vi "MainIdent RT.vi"   [LabVIEW 2018]
doc: "The myRIO Project template acquires acceleration data from the onboard accelerometer and displays the changes of acceleration values in a waveform chart."
uses:
  <vilib>/myRIO/Common/Instrument Driver Framework/myRIO v1.0/Encoder/typedefs/Encoder Signal Mode.ctl
  <vilib>/Platform/TimedLoop/XDataNode/timing_clust.ctl
  <vilib>/Platform/TimedLoop/XDataNode/nitl_modes.ctl
  <vilib>/Platform/TimedLoop/XDataNode/wakeup.ctl
  <vilib>/myRIO/Instrument Drivers/Onboard IO/AI/typedefs/AI Reference.ctl
  <vilib>/myRIO/Common/Instrument Driver Framework/Utilities/typedefs/myRIO Generic Hardware Reference.ctl
  <vilib>/myRIO/Common/Instrument Driver Framework/Utilities/typedefs/Hardware Version Enum.ctl
  <vilib>/myRIO/Common/Instrument Driver Framework/Utilities/typedefs/myRIO v1.0 Reference.ctl
  <vilib>/myRIO/Common/Instrument Driver Framework/Utilities/typedefs/Generic FPGA Reference.ctl
  <vilib>/myRIO/Common/Instrument Driver Framework/myRIO v1.0/AI/typedefs/AI Channels List.ctl
  <vilib>/myRIO/Common/Instrument Driver Framework/myRIO v1.0/AI/typedefs/AI Channels Enum.ctl
  <vilib>/myRIO/Common/Instrument Driver Framework/Utilities/typedefs/Analog Scaling Constants List.ctl
  <vilib>/myRIO/Common/Instrument Driver Framework/Utilities/typedefs/Analog Scaling Constants.ctl
  <vilib>/userdefined/High Color/nirio_resource_hc.ctl
  <vilib>/myRIO/Instrument Drivers/Onboard IO/PWM/typedefs/PWM Reference.ctl
  <vilib>/myRIO/Common/Instrument Driver Framework/myRIO v1.0/PWM/typedefs/PWM Channels Enum.ctl
  <vilib>/myRIO/Instrument Drivers/Onboard IO/PWM/typedefs/PWM Configuration.ctl
  <vilib>/myRIO/Common/Instrument Driver Framework/myRIO v1.0/Encoder/typedefs/Encoder Configuration v1.0.ctl
  <vilib>/myRIO/Instrument Drivers/Onboard IO/Encoder/typedefs/Encoder Reference.ctl
  <vilib>/myRIO/Common/Instrument Driver Framework/myRIO v1.0/Encoder/typedefs/Encoder Channels Enum.ctl
  <vilib>/myRIO/Common/Instrument Driver Framework/myRIO v1.0/AI/vis/myRIO v1.1 Open AI.vi
  <vilib>/myRIO/Common/Instrument Driver Framework/myRIO v1.0/PWM/vis/myRIO v1.1 Open PWM.vi
  <vilib>/myRIO/Common/Instrument Driver Framework/myRIO v1.0/Encoder/vis/myRIO v1.1 Open Encoder.vi
  <vilib>/myRIO/Common/Instrument Driver Framework/Utilities/vis/Validate Channels.vi
  <vilib>/myRIO/Common/Instrument Driver Framework/myRIO v1.0/AI/vis/myRIO v1.0 Reserve AI.vi
  <vilib>/myRIO/Common/Instrument Driver Framework/myRIO v1.0/PWM/vis/myRIO v1.0 Reserve PWM.vi
  <vilib>/myRIO/Instrument Drivers/Onboard IO/PWM/vis/Set Duty Cycle and Frequency.vi
  <vilib>/myRIO/Common/Instrument Driver Framework/myRIO v1.0/Encoder/vis/myRIO v1.0 Reserve Encoder.vi
  <vilib>/myRIO/Common/Instrument Driver Framework/myRIO v1.0/Encoder/vis/myRIO v1.0 Close Encoder.vi
  <vilib>/myRIO/Common/Instrument Driver Framework/myRIO v1.0/PWM/vis/myRIO v1.0 Close PWM.vi
  <vilib>/myRIO/Common/Instrument Driver Framework/myRIO v1.0/AI/vis/myRIO v1.0 Build MUX Configuration AI.vi
  <vilib>/myRIO/Common/Instrument Driver Framework/myRIO v1.0/Resource Manager/vis/myRIO v1.0 Reserve Channel List.vi
  <vilib>/myRIO/Common/Instrument Driver Framework/myRIO v1.0/PWM/vis/myRIO v1.0 Build MUX Configuration PWM.vi
  <vilib>/myRIO/Common/Instrument Driver Framework/myRIO v1.0/Encoder/vis/myRIO v1.0 Build MUX Configuration Encoder.vi
  <vilib>/myRIO/Common/Instrument Driver Framework/myRIO v1.0/Encoder/vis/myRIO v1.0 Unreserve Encoder.vi
  <vilib>/myRIO/Common/Instrument Driver Framework/myRIO v1.0/PWM/vis/myRIO v1.0 Unreserve PWM.vi
  <vilib>/myRIO/Common/Instrument Driver Framework/myRIO v1.0/Resource Manager/vis/myRIO v1.0 Reserve Channel.vi
  <vilib>/myRIO/Common/Instrument Driver Framework/myRIO v1.0/Resource Manager/vis/myRIO v1.0 Unreserve Channel.vi
  <vilib>/myRIO/Common/Instrument Driver Framework/myRIO v1.0/Resource Manager/vis/myRIO v1.0 Create Configuration List.vi
  <vilib>/myRIO/Common/Instrument Driver Framework/myRIO v1.0/Resource Manager/vis/myRIO v1.0 Unreserve Channel List.vi
  <vilib>/myRIO/Common/Instrument Driver Framework/myRIO v1.0/Resource Manager/vis/myRIO v1.0 Build Mutex Name.vi
  <vilib>/Utility/VariantDataType/GetNumericInfo.vi
  <vilib>/Utility/error.llb/Error Cluster From Error Code.vi
  <vilib>/myRIO/Common/Instrument Driver Framework/myRIO v1.0/myRIO v1.1 Open.vi
  <vilib>/myRIO/Common/Instrument Driver Framework/Utilities/vis/IO Manager.vi
  <vilib>/myRIO/Common/Instrument Driver Framework/Utilities/vis/Configuration Manager.vi
  <vilib>/myRIO/Common/Instrument Driver Framework/myRIO v1.0/Resource Manager/vis/myRIO v1.0 Configure IO.vi
  <vilib>/myRIO/Common/Instrument Driver Framework/myRIO v1.0/myRIO v1.0 Close.vi
  <vilib>/myRIO/Common/Instrument Driver Framework/myRIO v1.0/PWM/vis/myRIO v1.0 Write PWM.vi
  <vilib>/myRIO/Common/Instrument Driver Framework/myRIO v1.0/Encoder/vis/myRIO v1.0 Configure Encoder.vi
  <vilib>/myRIO/Common/Instrument Driver Framework/myRIO v1.0/Encoder/vis/myRIO v1.0 Enable Encoder.vi
  <vilib>/myRIO/Common/Instrument Driver Framework/myRIO v1.0/AI/vis/myRIO v1.0 Get Scaling Constants AI.vi
  <vilib>/myRIO/Common/Instrument Driver Framework/myRIO v1.0/AI/vis/myRIO v1.0 Read AI.vi
  <vilib>/myRIO/Common/Instrument Driver Framework/myRIO v1.0/Encoder/vis/myRIO v1.0 Read Encoder.vi
  <vilib>/myRIO/Common/Instrument Driver Framework/myRIO v1.0/Encoder/vis/myRIO v1.0 Shutdown Encoder.vi
  <vilib>/myRIO/Common/Instrument Driver Framework/myRIO v1.0/PWM/vis/myRIO v1.0 Shutdown PWM.vi
  <vilib>/platform/TimedLoop/XDataNode/XDataNode.xnode
  <vilib>/myRIO/Instrument Drivers/Onboard IO/PWM/vis/myRIO PWM Open.xnode
  <vilib>/myRIO/Instrument Drivers/Onboard IO/Encoder/vis/myRIO Encoder Open.xnode
  <vilib>/myRIO/Instrument Drivers/Onboard IO/AI/vis/myRIO AI Open.xnode
  <vilib>/Platform/TimedLoop/XDataNode/XDNodeRunTimeDep.lvlib
  <vilib>/myRIO/Instrument Drivers/Onboard IO/Encoder/Encoder.lvlib
  <vilib>/myRIO/Instrument Drivers/Onboard IO/PWM/PWM.lvlib
  <vilib>/myRIO/Instrument Drivers/Onboard IO/AI/AI.lvlib
types:
  T1 = typedef "Encoder Signal Mode.ctl" = enum16{"Quadrature phase signal", "Step and direction signal"}
  T2 = typedef "AI.lvlib/AI Reference.ctl" = cluster{"myRIO Reference":T3, "AI Channels List":T7, "AI Scaling Constants List":T9}
  T3 = typedef "myRIO Generic Hardware Reference.ctl" = cluster{"myRIO Model":T4, "myRIO Hardware Reference":T5}
  T4 = typedef "Hardware Version Enum.ctl" = enum16{"Unknown", "myRIO-1900", "myRIO-1950", "roboRIO", "NI ELVIS RIO CM", "ELVIS III"}
  T5 = typedef "myRIO v1.0 Reference.ctl" = cluster{"Generic FPGA Reference":T6, "Allow multiple opens":bool}
  T6 = typedef "Generic FPGA Reference.ctl" = refnum<k20>
  T7 = typedef "AI Channels List.ctl" = T8[]
  T8 = typedef "AI Channels Enum.ctl" = enum16{"Not Connected", "AudioIn/Left", "AudioIn/Right", "C/AI0", "C/AI1", "A/AI0", "A/AI1", "A/AI2", "A/AI3", "A/AI4", "A/AI5", "A/AI6", "A/AI7", "B/AI0", "B/AI1", "B/AI2", "B/AI3", "B/AI4", "B/AI5", "B/AI6", "B/AI7", "AI/AI0", "AI/AI1", "AI/AI2", "AI/AI3", "A/AI0 (DIFF)", "A/AI1 (DIFF)", "A/AI2 (DIFF)", "A/AI3 (DIFF)", "B/AI0 (DIFF)", "B/AI1 (DIFF)", "B/AI2 (DIFF)", "B/AI3 (DIFF)"}
  T9 = typedef "Analog Scaling Constants List.ctl" = T10[]
  T10 = typedef "Analog Scaling Constants.ctl" = cluster{"LSB Weight (Volts)":dbl, "Offset (Volts)":dbl, "Signed?":bool}
  T11 = typedef "PWM.lvlib/PWM Reference.ctl" = cluster{"myRIO Reference":T3, "PWM Channels Enum":T12, "PWM Configuration":T13}
  T12 = typedef "PWM Channels Enum.ctl" = enum16{"Not Connected", "C/PWM0", "C/PWM1", "A/PWM0", "A/PWM1", "A/PWM2", "A/PWM3", "A/PWM4", "A/PWM5", "A/PWM6", "A/PWM7", "A/PWM8", "A/PWM9", "A/PWM10", "A/PWM11", "A/PWM12", "A/PWM13", "A/PWM14", "A/PWM15", "A/PWM16", "A/PWM17", "A/PWM18", "A/PWM19", "B/PWM0", "B/PWM1", "B/PWM2", "B/PWM3", "B/PWM4", "B/PWM5", "B/PWM6", "B/PWM7", "B/PWM8", "B/PWM9", "B/PWM10", "B/PWM11", "B/PWM12", "B/PWM13", "B/PWM14", "B/PWM15", "B/PWM16", "B/PWM17", "B/PWM18", "B/PWM19", "PWM/PWM0", "PWM/PWM1", "PWM/PWM2", "PWM/PWM3", "PWM/PWM4", "PWM/PWM5", "PWM/PWM6", "PWM/PWM7", "PWM/PWM8", "PWM/PWM9"}
  T13 = typedef "PWM.lvlib/PWM Configuration.ctl" = cluster{"Frequency":dbl, "Duty Cycle":dbl}
  T14 = typedef "Encoder.lvlib/Encoder Reference.ctl" = cluster{"myRIO Reference":T3, "Encoder Channels Enum":T15}
  T15 = typedef "Encoder Channels Enum.ctl" = enum16{"Not Connected", "C/ENC0", "C/ENC1", "A/ENC", "A/ENC0", "A/ENC1", "A/ENC2", "A/ENC3", "A/ENC4", "A/ENC5", "A/ENC6", "A/ENC7", "A/ENC8", "A/ENC9", "B/ENC", "B/ENC0", "B/ENC1", "B/ENC2", "B/ENC3", "B/ENC4", "B/ENC5", "B/ENC6", "B/ENC7", "B/ENC8", "B/ENC9", "DIO/ENC0", "DIO/ENC1", "DIO/ENC2", "DIO/ENC3", "DIO/ENC4"}
  T16 = typedef "XDNodeRunTimeDep.lvlib/timing_clust.ctl" = cluster{"Expected End [f-1]":u64, "Actual End [f-1]":u64, "Finished Late? [f-1]":bool, "Expected End [i-1]":u64, "Actual End [i-1]":u64, "Finished Late? [i-1]":bool, "Expected Start [i]":u64, "Actual Start [i]":u64, "Expected Start [f]":u64, "Actual Start [f]":u64, "Source Name":string, "Structure Name":string, "Period":i64, "Deadline":i64, "Offset":i64, "Start":i64, "Priority":i32, "Timeout":i32, "Mode":T17, "Wakeup Reason":T18, "Error":errorcluster, "Source Type":string, "Secondary Source Type":string, "Global End Time":u64, "Global Start Time":u64, "Frame Duration":u64, "Iteration Duration":u64, "Assigned CPU":i32, "I/O Scan Engine Mode":u32}
  T17 = typedef "XDNodeRunTimeDep.lvlib/nitl_modes.ctl" = enum32{"No Change", "Process missed periods, maintain original phase", "Discard missed periods, maintain original phase", "Process missed periods, ignore original phase", "Discard missed periods, ignore original phase"}
  T18 = typedef "XDNodeRunTimeDep.lvlib/wakeup.ctl" = enum32{"Normal", "Aborted", "Asynchronous wakeup", "Timing source error", "Timed loop error", "Timeout"}
  T19 = cluster{"dbl Scaled Value":dbl, dbl, "Double":dbl, "seconds since 1Jan1904":timestamp}
  T20 = cluster{"Double":dbl, "dbl Scaled Value":dbl, "Output":dbl, "seconds since 1Jan1904":timestamp}
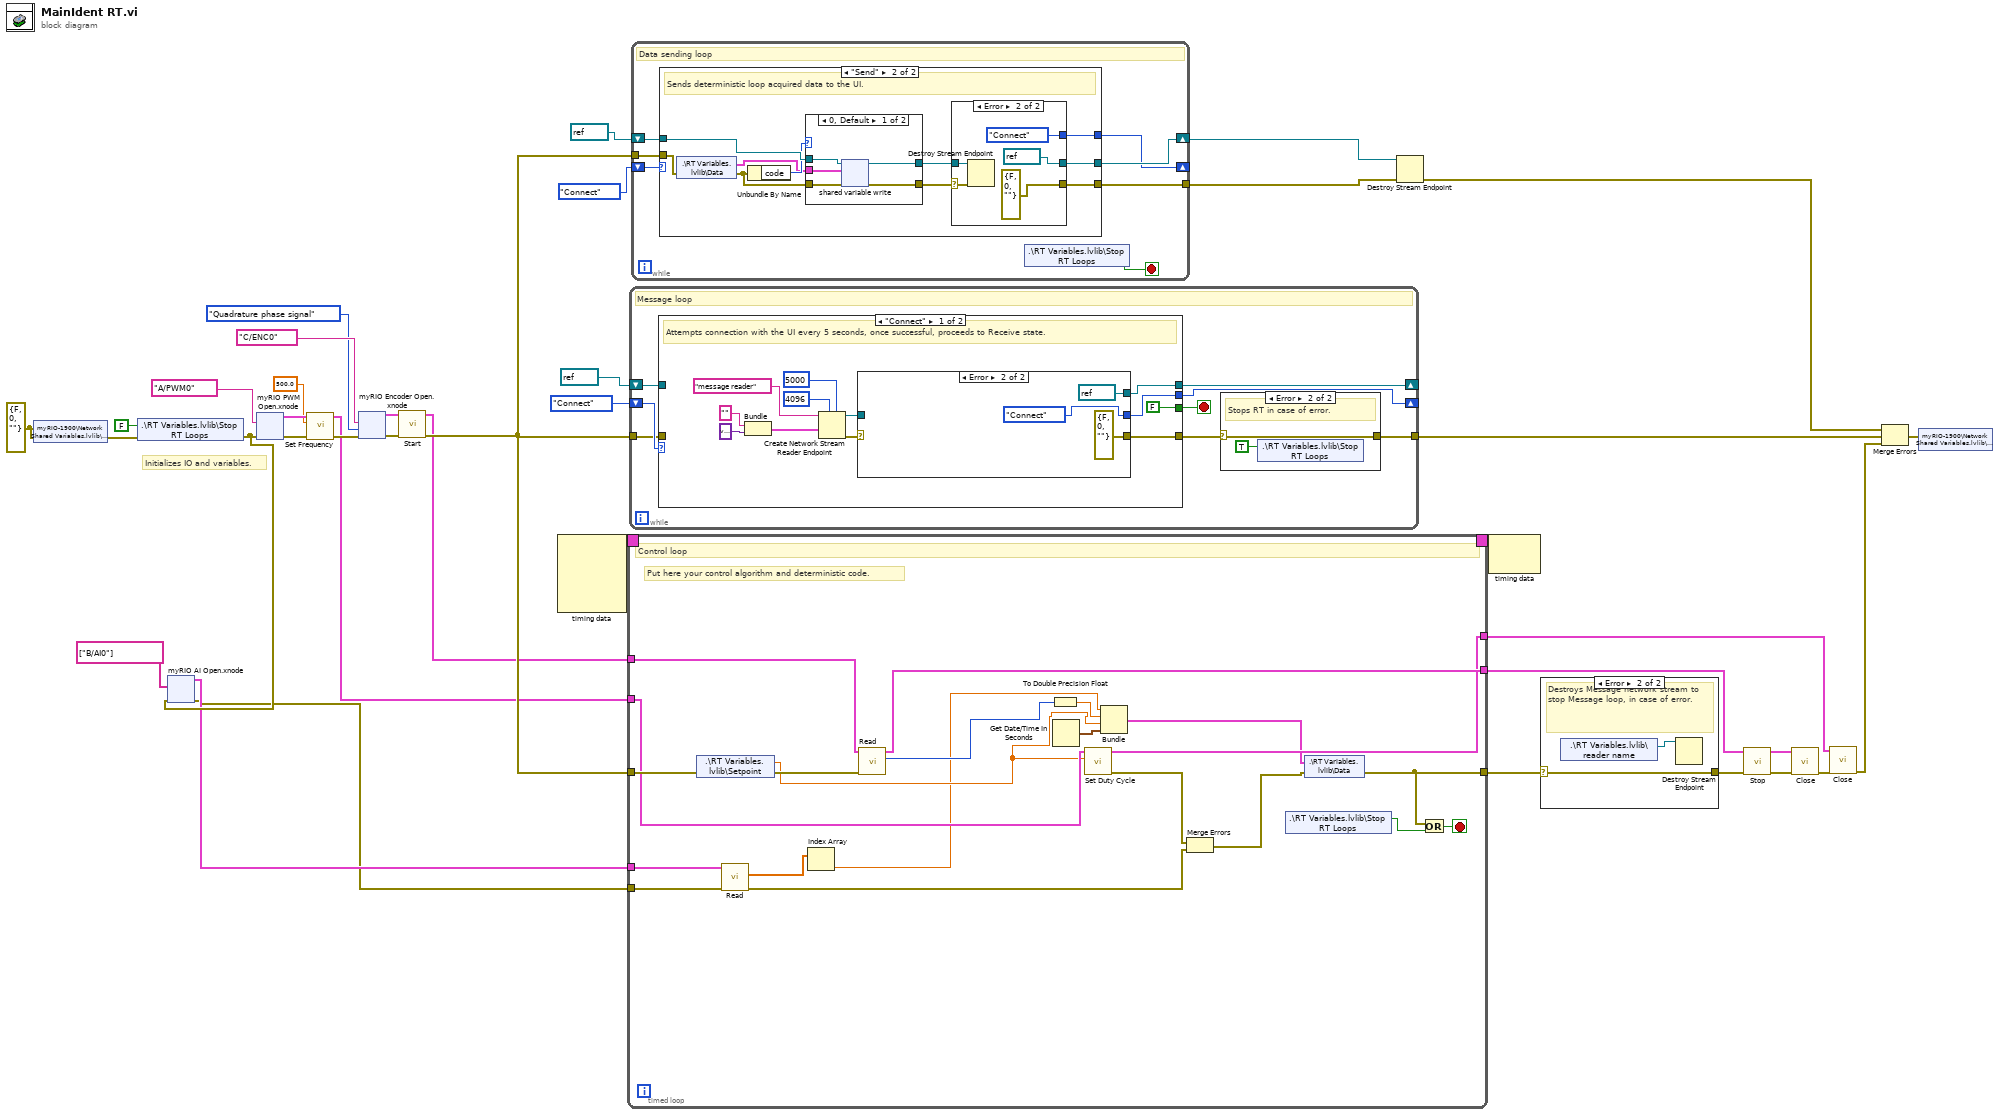
[diagram p0: block diagram]
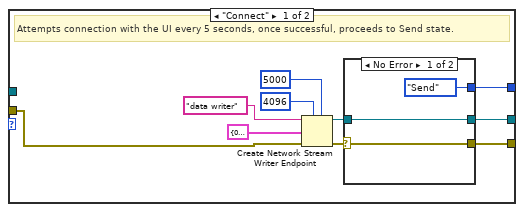
[diagram p3: hidden frame]
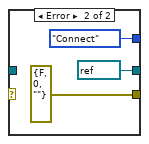
[diagram p4: hidden frame]
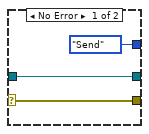
[diagram p5: hidden frame]
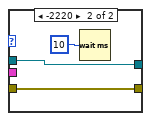
[diagram p6: hidden frame]
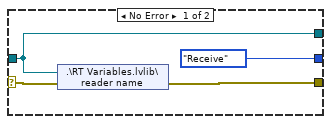
[diagram p8: hidden frame]
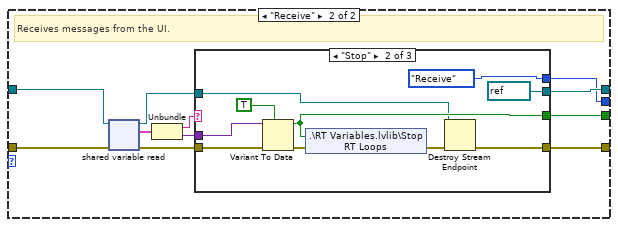
[diagram p9: hidden frame]
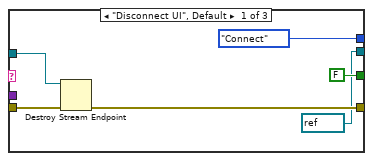
[diagram p10: hidden frame]
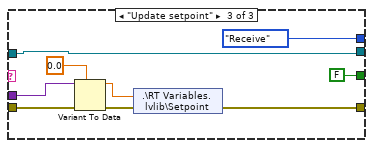
[diagram p11: hidden frame]
diagram:
  w25 = errorcluster {"status"=FALSE, "code"=0, "source"=""} ("error IO")
  # "Initializes IO and variables."
  n1 = shared-variable "myRIO-1900\\Network Shared Variables.lvlib\\error IO"(w25, error in=w25) -> (error out=w26:errorcluster)
  n2 = shared-variable ".\\RT Variables.lvlib\\Stop RT Loops"(FALSE ("Stop RT Loops"), error in=w26) -> (error out=w3:errorcluster)
  n3 = xnode "myRIO AI Open.xnode"("error in (no error)"=w3, "Channel Names"=tag[] ["B/AI0"]) -> ("error out"=w1:errorcluster, "AI Ref Out"=w2:T2)  [unwired: 1 in]
  n4 = xnode "myRIO PWM Open.xnode"("error in (no error)"=w3, "Channel Name"=tag "A/PWM0") -> ("error out"=w13:errorcluster, "PWM Ref Out"=w12:T11)  [unwired: 1 in]
  n5 = call <vilib>:"Set Frequency.vi"("error in (no error)"=w13, "Frequency [Hz]"=500.0, "PWM Ref In"=w12) -> ("error out"=w11:errorcluster, "PWM Ref Out"=w8:T11)  [unwired: 6 in]
  n6 = xnode "myRIO Encoder Open.xnode"("error in (no error)"=w11, "Channel Name"=tag "C/ENC0", "Encoder Signal Mode"=Encoder_Signal_Mode."Quadrature phase signal") -> ("error out"=w22:errorcluster, "Encoder Ref Out"=w21:T14)  [unwired: 2 in]
  n7 = call <vilib>:"Start.vi"("error in (no error)"=w22, "Encoder Ref In"=w21) -> ("error out"=w19:errorcluster, "Encoder Ref Out"=w18:T14)  [unwired: 8 in]
  n8 = node-c288() -> (w38:T16)  [unwired: 4 in]
  n9 = timed-loop {
    timing: w38 -> [_]
    timing-out: [_] -> w37
    tunnel: w19 -> [w58]
    tunnel: [w54] -> w24
    tunnel: w18 -> [w53]
    tunnel: [w52] -> w14
    tunnel: w8 -> [w51]
    tunnel: [w48] -> w7
    tunnel: w2 -> [w45]
    tunnel: w1 -> [w44]
    stop <- w55 stop-if-true
    # "Put here your control algorithm and deterministic code."
    # "Control loop"
    n10 = shared-variable ".\\RT Variables.lvlib\\Setpoint"(error in=w58) -> (w46:dbl, error out=w59:errorcluster)
    n11 = call <vilib>:"Read.vi"("error in (no error)"=w44, "AI Ref In"=w45) -> ("error out"=w39:errorcluster, "Values"=w43:dbl[])  [unwired: 7 in, 1 out]
    n12 = Index Array(array=w43) -> (element=w42:dbl)  [unwired: 1 in]
    n13 = call <vilib>:"Read.vi"("error in (no error)"=w59, "Encoder Ref In"=w53) -> ("Counter Value"=w50:i32, "Encoder Ref Out"=w52:T14)  [unwired: 5 in, 3 out]
    n14 = To Double Precision Float(number=w50) -> (double precision float=w49:dbl)
    n15 = Get Date/Time In Seconds() -> (seconds since 1Jan1904=w57:timestamp)
    n16 = call <vilib>:"Set Duty Cycle.vi"("Duty Cycle"=w46, "PWM Ref In"=w51) -> ("error out"=w40:errorcluster, "PWM Ref Out"=w48:T11)  [unwired: 7 in]
    n17 = Bundle("dbl Scaled Value"=w42, w49, "Double"=w46, "seconds since 1Jan1904"=w57) -> (w47:T19)  [unwired: 1 in]
    n18 = Merge Errors(w40, w39) -> (w41:errorcluster)
    n19 = shared-variable ".\\RT Variables.lvlib\\Stop RT Loops"() -> (w56:bool)  [unwired: 1 in, 1 out]
    n20 = shared-variable ".\\RT Variables.lvlib\\Data"(w47, error in=w41) -> (error out=w54:errorcluster)
    n21 = Or(x=w54, y=w56) -> (x .or. y?=w55:bool)
  }
  n22 = while {
    tunnel: [w62] -> w28
    shift-right: [w68] -> _
    shift-left: refnum<k21> refnum ("reader name") -> [w66]
    shift-right: [w67] -> _
    shift-left: enum16{"Connect", "Receive"}."Connect" ("Message states") -> [w69]
    tunnel: w19 -> [w64]
    stop <- w65 stop-if-true
    # "Message loop"
    n23 = case shown="\"Connect\"" w69 {
      tunnel: [w75 w95] -> w63
      tunnel: [w74 w97] -> w68
      tunnel: [w82 w92] -> w67
      tunnel: w66 -> [_ w102]
      tunnel: w64 -> [_ w94]
      tunnel: [FALSE ("Stop RT Loops") w93] -> w65
      frame "Connect" {
        # "Attempts connection with the UI every 5 seconds, once successful, proceeds to Receive state."
        n24 = Bundle("", variant) -> (w78:cluster{string, variant})  [unwired: 1 in]
        n25 = Create Network Stream Reader Endpoint(5:5000 ("timeout in ms (-1)"), 7:4096 ("reader buffer size"), 9:w78, 11:"message reader" ("reader name")) -> (0:w77:errorcluster, 3:w73:refnum<k21>)  [unwired: 3 in]
        n26 = case shown="Error" w77 {
          selector: w77 -> [w86 _]
          tunnel: [enum16{"Connect", "Receive"}."Receive" ("Message states") enum16{"Connect", "Receive"}."Connect" ("Message states")] -> w82
          tunnel: [w85 errorcluster {"status"=FALSE, "code"=0, "source"=""} ("error IO")] -> w75
          tunnel: [w87 refnum<k21> refnum ("reader name")] -> w74
          tunnel: w73 -> [w87 _]
          frame No Error {
            n27 = shared-variable ".\\RT Variables.lvlib\\reader name"(w87, error in=w86) -> (error out=w85:errorcluster)
          }
          frame Error {
          }
        }
      }
      frame "Receive" {
        # "Receives messages from the UI."
        n28 = shared-variable-read(w102, w94) -> (w96:refnum<k21>, w98:errorcluster, w101:cluster{string, variant})  [unwired: 1 in, 1 out]
        n29 = Unbundle(w101) -> (w100:string, w99:variant)
        n30 = case shown="\"Stop\"" w100 {
          tunnel: w99 -> [_ w116 w127]
          tunnel: w98 -> [w106 w118 w126]
          tunnel: [w105 w112 w122] -> w95
          tunnel: [refnum<k21> refnum ("reader name") refnum<k21> refnum ("reader name") w121] -> w97
          tunnel: w96 -> [w104 w111 w121]
          tunnel: [FALSE ("Stop RT Loops") w115 FALSE ("Stop RT Loops")] -> w93
          tunnel: [enum16{"Connect", "Receive"}."Connect" ("Message states") enum16{"Connect", "Receive"}."Receive" ("Message states") enum16{"Connect", "Receive"}."Receive" ("Message states")] -> w92
          frame "Disconnect UI", Default {
            n31 = Destroy Stream Endpoint(8:w106, 11:w104) -> (0:w105:errorcluster)
          }
          frame "Stop" {
            n32 = Variant To Data(error in=w118, type=TRUE ("Stop RT Loops"), Variant=w116) -> (data=w115:bool, error out=w117:errorcluster)
            n33 = shared-variable ".\\RT Variables.lvlib\\Stop RT Loops"(w115, error in=w117) -> (error out=w113:errorcluster)
            n34 = Destroy Stream Endpoint(8:w113, 11:w111) -> (0:w112:errorcluster)
          }
          frame "Update setpoint" {
            n35 = Variant To Data(error in=w126, type=0.0, Variant=w127) -> (data=w124:dbl, error out=w123:errorcluster)
            n36 = shared-variable ".\\RT Variables.lvlib\\Setpoint"(w124, error in=w123) -> (error out=w122:errorcluster)
          }
        }
      }
    }
    n37 = case shown="Error" w63 {
      selector: w63 -> [w70 w71]
      tunnel: [w70 w71] -> w62
      frame No Error {
        # "No action required."
      }
      frame Error {
        # "Stops RT in case of error."
        n38 = shared-variable ".\\RT Variables.lvlib\\Stop RT Loops"(TRUE ("Stop RT Loops")) -> ()  [unwired: 1 in, 1 out]
      }
    }
  }
  n39 = while {
    shift-right: [w132] -> w31
    shift-left: refnum<k21> refnum ("writer endpoint") -> [w130]
    tunnel: [w131] -> w32
    tunnel: w19 -> [w129]
    shift-right: [w128] -> _
    shift-left: enum16{"Connect", "Send"}."Connect" ("Message states") -> [w133]
    stop <- w134 stop-if-true
    # "Data sending loop"
    n40 = case shown="\"Send\"" w133 {
      tunnel: [w137 w153] -> w131
      tunnel: [w135 w151] -> w132
      tunnel: [w142 w154] -> w128
      tunnel: w130 -> [_ w160]
      tunnel: w129 -> [w138 w159]
      frame "Connect" {
        # "Attempts connection with the UI every 5 seconds, once successful, proceeds to Send state."
        n41 = Create Network Stream Writer Endpoint(5:5000 ("timeout in ms (-1)"), 7:4096 ("writer buffer size"), 8:w138, 9:T20 {"Double"=0.0, "dbl Scaled Value"=0.0, "Output"=0.0, "seconds since 1Jan1904"=timestamp(0 s since 1904-01-01)} ("Data"), 11:"data writer" ("writer name")) -> (0:w140:errorcluster, 3:w136:refnum<k21>)  [unwired: 2 in]
        n42 = case shown="No Error" w140 {
          selector: w140 -> [w145 _]
          tunnel: [enum16{"Connect", "Send"}."Send" ("Message states") enum16{"Connect", "Send"}."Connect" ("Message states")] -> w142
          tunnel: [w145 errorcluster {"status"=FALSE, "code"=0, "source"=""} ("error IO")] -> w137
          tunnel: w136 -> [w147 _]
          tunnel: [w147 refnum<k21> refnum ("writer endpoint")] -> w135
          frame No Error {
          }
          frame Error {
          }
        }
      }
      frame "Send" {
        # "Sends deterministic loop acquired data to the UI."
        n43 = shared-variable ".\\RT Variables.lvlib\\Data"(error in=w159) -> (w156:T20, error out=w158:errorcluster)
        n44 = Unbundle By Name(w158) -> ("code"=w157:i32)
        n45 = case shown="0, Default" w157 {
          tunnel: [w173 w175] -> w155
          tunnel: [w172 w174] -> w152
          tunnel: w160 -> [w171 w174]
          tunnel: w158 -> [w170 w175]
          tunnel: w156 -> [w169 _]
          frame 0, Default {
            n46 = shared-variable-write(w171, w170, w169) -> (w172:refnum<k21>, w173:errorcluster)  [unwired: 1 in, 1 out]
          }
          frame -2220 {
            n47 = Wait (ms)(milliseconds to wait=u32 10) -> ()  [unwired: 1 out]
          }
        }
        n48 = case shown="Error" w155 {
          selector: w155 -> [w163 w167]
          tunnel: [enum16{"Connect", "Send"}."Send" ("Message states") enum16{"Connect", "Send"}."Connect" ("Message states")] -> w154
          tunnel: [w163 errorcluster {"status"=FALSE, "code"=0, "source"=""} ("error IO")] -> w153
          tunnel: w152 -> [w161 w166]
          tunnel: [w161 refnum<k21> refnum ("writer endpoint")] -> w151
          frame No Error {
          }
          frame Error {
            n49 = Destroy Stream Endpoint(8:w167, 11:w166) -> ()  [unwired: 1 out]
          }
        }
      }
    }
    n50 = shared-variable ".\\RT Variables.lvlib\\Stop RT Loops"() -> (w134:bool)  [unwired: 1 in, 1 out]
  }
  n51 = Destroy Stream Endpoint(8:w32, 11:w31) -> (0:w29:errorcluster)
  n52 = node-c288(w37) -> ()  [unwired: 1 out]
  n53 = case shown="Error" w24 {
    selector: w24 -> [w177 w178]
    tunnel: [w177 w178] -> w15
    frame No Error {
      # "No action required."
    }
    frame Error {
      # "Destroys Message network stream to stop Message loop, in case of error."
      n54 = shared-variable ".\\RT Variables.lvlib\\reader name"() -> (w179:refnum<k21>)  [unwired: 1 in, 1 out]
      n55 = Destroy Stream Endpoint(11:w179) -> ()  [unwired: 1 in, 1 out]
    }
  }
  n56 = call <vilib>:"Stop.vi"("error in (no error)"=w15, "Encoder Ref In"=w14) -> ("error out"=w16:errorcluster, "Encoder Ref Out"=w17:T14)  [unwired: 8 in]
  n57 = call <vilib>:"Close.vi"("error in (no error)"=w16, "Encoder Ref In"=w17) -> ("error out"=w10:errorcluster)  [unwired: 9 in]
  n58 = call <vilib>:"Close.vi"("error in (no error)"=w10, "PWM Ref In"=w7) -> ("error out"=w9:errorcluster)  [unwired: 9 in]
  n59 = Merge Errors(w29, w28, w9) -> (w27:errorcluster)
  n60 = shared-variable "myRIO-1900\\Network Shared Variables.lvlib\\error IO"(w27) -> ()  [unwired: 1 in, 1 out]
